vi "R1NH4SignalProcess.vi"(9 "error":errorcluster, 11 "LabVIEW Web Service":refnum<class "Web Service.lvclass">) -> (1 "error out":errorcluster)   [LabVIEW 2016]
uses:
  <vilib>/wsapi/Web Service.lvclass
  Controls/Tri State Control.ctl
  Controls/ISE_CF.ctl
panel:
  out "R1Na":T2 {"Steady State?" items=["False", "True", "NaN", ""]}
  out "Carousel Array":dbl[][](array[numeric])
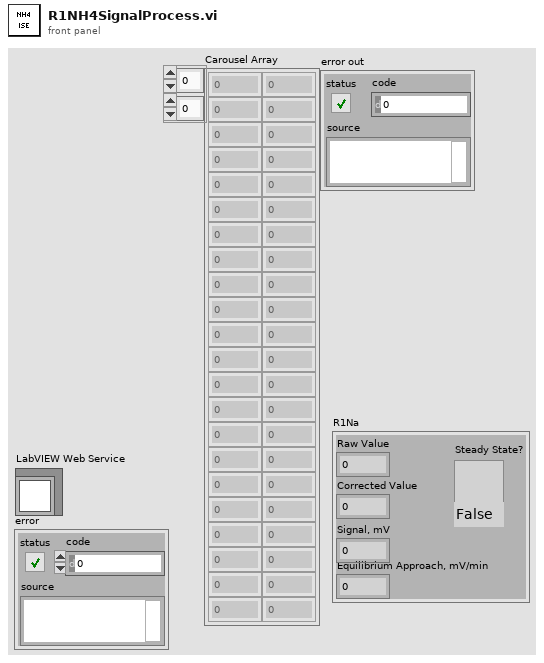
[diagram p1: front panel]
types:
  T1 = typedef "Tri State Control.ctl" = u16
  T2 = cluster{"Raw Value":dbl, "Corrected Value":dbl, "Signal, mV":dbl, "Equilibrium Approach, mV/min":dbl, "Steady State?":T1}
  T3 = typedef "ISE_CF.ctl" = cluster{"Correction Factor":dbl, "Ion":string, "Correct For Ion?":bool}
  T4 = cluster{"Equil Approach Set point, mV/min":dbl, "Equil Approach dt, s":dbl, "Interference Correction Factors":T3[], "Detect Equilibrium?":bool, "Probe Intercept":dbl, "Probe Slope":dbl, "Baseline":dbl, "Detection Limit, M":dbl}
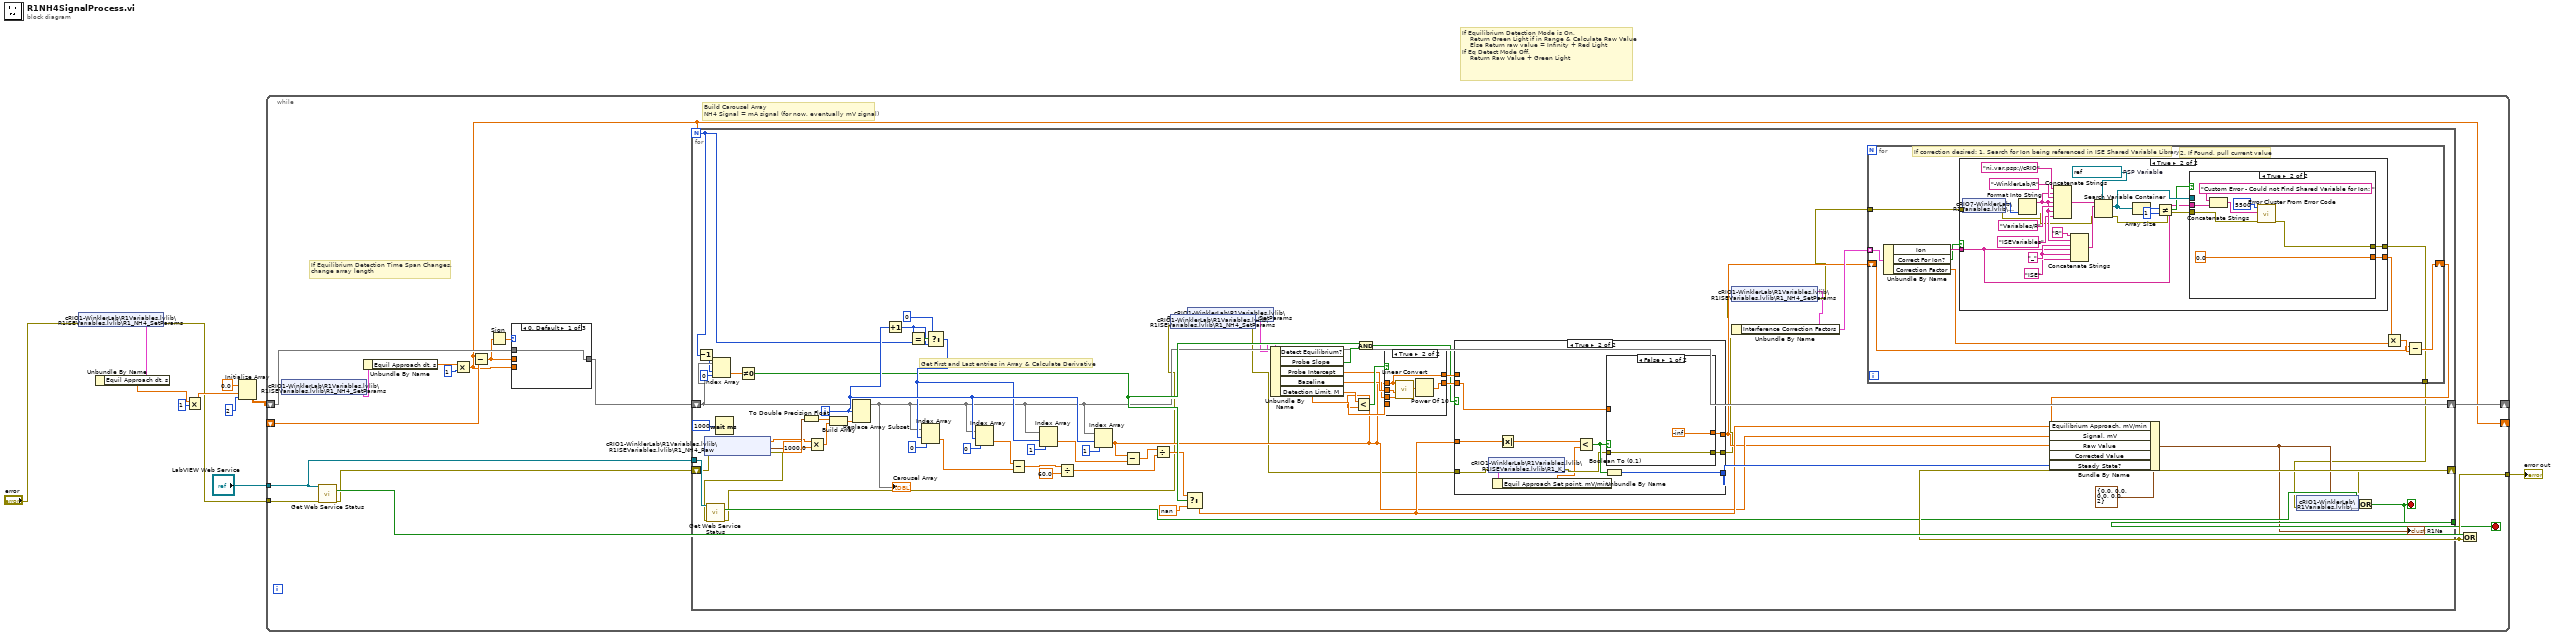
[diagram p0: block diagram]
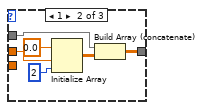
[diagram p2: hidden frame]
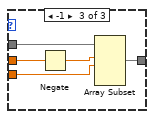
[diagram p3: hidden frame]
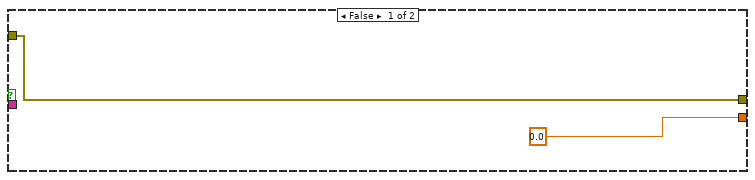
[diagram p4: hidden frame]
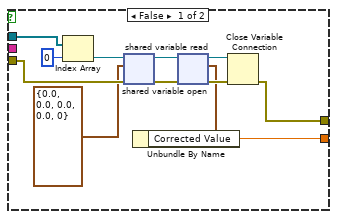
[diagram p5: hidden frame]
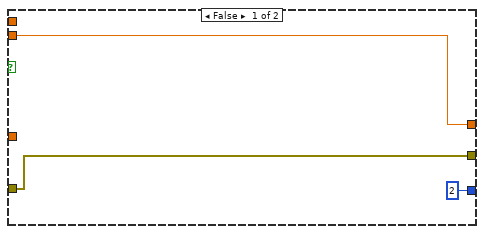
[diagram p7: hidden frame]
diagram:
  # "If Equilibrium Detection Mode is On, \n    Return Green Light if in Range & Calculate Raw Value\n    Else Return raw value = Infinity + Red Light\nIf Eq Detect Mode Off,\n    Return Raw Value + Green Light"
  n1 = shared-variable "cRIO1-WinklerLab\\R1Variables.lvlib\\R1ISEVariables.lvlib\\R1_NH4_SetParams"(error in="error") -> (w5:T4, error out=w1:errorcluster)
  n2 = Unbundle By Name(w5) -> ("Equil Approach dt, s"=w4:dbl)
  n3 = Multiply(x=w4, y=1) -> (x*y=w3:dbl)
  n4 = Initialize Array(0.0 ("element"), w3, 2 ("dimension size")) -> (w7:dbl[][])
  n5 = while {
    tunnel: "LabVIEW Web Service" -> [w27]
    tunnel: w1 -> [w18]
    shift-right: [w21] -> _
    shift-left: w7 -> [w24]
    shift-right: [w12] -> _
    shift-left: _ -> [w20]
    tunnel: [w17] -> w6
    stop <- w16 stop-if-true
    # "Build Carousel Array\nNH4 Signal = mA signal (for now, eventually mV signal)"
    # "If Equilibrium Detection Time Span Changes, \nchange array length"
    n6 = shared-variable "cRIO1-WinklerLab\\R1Variables.lvlib\\R1ISEVariables.lvlib\\R1_NH4_SetParams"() -> (w13:T4)  [unwired: 1 in, 1 out]
    n7 = call <vilib>:"Get Web Service Status.vi"("LabVIEW Web Service"=w27, "error in (no error)"=w18) -> ("service stopping?"=w19:bool, "error out"=w15:errorcluster)  [unwired: 11 in, 1 out]
    n8 = Unbundle By Name(w13) -> ("Equil Approach dt, s"=w14:dbl)
    n9 = Multiply(x=w14, y=1) -> (x*y=w12:dbl)
    n10 = Subtract(x=w12, y=w20) -> (x-y=w23:dbl)
    n11 = Sign(1:w23) -> (0:w25:dbl)
    n12 = case shown="0, Default" w25 {
      tunnel: w24 -> [w28 w32 w35]
      tunnel: w23 -> [_ w29 w37]
      tunnel: [w28 w30 w39] -> w22
      tunnel: w12 -> [_ _ w38]
      frame 0, Default {
      }
      frame 1 {
        n13 = Initialize Array(0.0 ("element"), w29, 2 ("dimension size")) -> (w31:dbl[][])
        n14 = Build Array (concatenate)(w32, w31) -> (w30:dbl[][])
      }
      frame -1 {
        n15 = Negate(x=w37) -> (-x=w36:dbl)
        n16 = Array Subset(array=w35, index (row)=w36, length (row)=w38) -> (w39:dbl[][])  [unwired: 2 in]
      }
    }
    n17 = for {
      N: w12 -> [w79]
      tunnel: w27 -> [w101]
      shift-right: [w74] -> w21
      shift-left: w22 -> [w85]
      shift-right: [w51] -> w17
      shift-left: w15 -> [w67]
      tunnel: [w66] -> w16
      i -> [w90]
      stop <- w66 stop-if-true
      # "Get First and Last entries in Array & Calculate Derivative"
      n18 = Decrement(x=w79) -> (x-1=w80:i32)
      n19 = shared-variable "cRIO1-WinklerLab\\R1Variables.lvlib\\R1ISEVariables.lvlib\\R1_NH4_Raw"(error in=w67) -> (w63:dbl, error out=w76:errorcluster, w77:timestamp)
      n20 = call <vilib>:"Get Web Service Status.vi"("LabVIEW Web Service"=w101, "error in (no error)"=w76) -> ("service stopping?"=w78:bool, "error out"=w43:errorcluster)  [unwired: 11 in, 1 out]
      n21 = Index Array(array=w85, index (row)=w80, index (col)=0 ("disabled index (col)")) -> (element=w83:dbl)
      n22 = Wait (ms)(milliseconds to wait=u32 1000) -> ()  [unwired: 1 out]
      n23 = Not Equal To 0?(x=w83) -> (x != 0?=w82:bool)
      n24 = To Double Precision Float(number=w77) -> (double precision float=w100:dbl)
      n25 = Multiply(x=w63, y=1000.0) -> (x*y=w62:dbl)
      n26 = Build Array(w100, w62) -> (w99:dbl[])
      n27 = Replace Array Subset(array=w85, new element=w99, index (row)=w90) -> (w74:dbl[][])  [unwired: 1 in]
      "Carousel Array" <- w74
      n28 = Increment(x=w90) -> (x+1=w60:i32)
      n29 = Equal?(x=w60, y=w79) -> (x = y?=w87:bool)
      n30 = Select(t=0, s=w87, f=w60) -> (s? t:f=w86:i32)
      n31 = Index Array(array=w74, index (row)=w86, index (col)=0 ("disabled index (col)")) -> (element=w92:dbl)
      n32 = Index Array(array=w74, index (row)=w90, index (col)=0 ("disabled index (col)")) -> (element=w88:dbl)
      n33 = Subtract(x=w88, y=w92) -> (x-y=w57:dbl)
      n34 = Index Array(array=w74, index (row)=w86, index (col)=1 ("disabled index (col)")) -> (element=w91:dbl)
      n35 = Divide(x=w57, y=60.0) -> (x/y=w56:dbl)
      n36 = Index Array(array=w74, index (row)=w90, index (col)=1 ("disabled index (col)")) -> (element=w52:dbl)
      n37 = Subtract(x=w52, y=w91) -> (x-y=w97:dbl)
      n38 = Divide(x=w97, y=w56) -> (x/y=w73:dbl)
      n39 = shared-variable "cRIO1-WinklerLab\\R1Variables.lvlib\\R1ISEVariables.lvlib\\R1_NH4_SetParams"(error in=w43) -> (w45:T4, error out=w44:errorcluster)
      n40 = Select(t=w73, s=w82, f=nan) -> (s? t:f=w54:dbl)
      n41 = shared-variable "cRIO1-WinklerLab\\R1Variables.lvlib\\R1ISEVariables.lvlib\\R1_NH4_SetParams"() -> ()  [unwired: 1 in, 2 out]
      n42 = Unbundle By Name(w45) -> ("Detect Equilibrium?"=w75:bool, "Probe Slope"=w71:dbl, "Probe Intercept"=w53:dbl, "Baseline"=w61:dbl, "Detection Limit, M"=w65:dbl)
      n43 = Less?(x=w61, y=w52) -> (x < y?=w72:bool)
      n44 = And(x=w82, y=w75) -> (x .and. y?=w68:bool)
      n45 = case shown="True" w72 {
        tunnel: w71 -> [_ w161]
        tunnel: w53 -> [_ w160]
        tunnel: w52 -> [w156 w159]
        tunnel: [w155 w158] -> w70
        tunnel: [w156 w159] -> w69
        tunnel: w65 -> [w155 _]
        frame False {
        }
        frame True {
          n46 = call "Linear Convert.vi"("Intercept"=w160, "Slope"=w161, "Signal"=w159) -> ("Result"=w157:dbl)  [unwired: 8 in]
          n47 = Power Of 10(x=w157) -> (10^x=w158:dbl)
        }
      }
      n48 = case shown="True" w68 {
        tunnel: [w164 w175] -> w48
        tunnel: w54 -> [_ w174]
        tunnel: [i16 2 w172] -> w89
        tunnel: w44 -> [w163 w168]
        tunnel: [w163 w169] -> w42
        tunnel: w70 -> [w164 w170]
        tunnel: w69 -> [_ _]
        frame False {
        }
        frame True {
          n49 = shared-variable "cRIO1-WinklerLab\\R1Variables.lvlib\\R1ISEVariables.lvlib\\R1_K_SetParams"(error in=w168) -> (w165:T4, error out=w167:errorcluster)
          n50 = Unbundle By Name(w165) -> ("Equil Approach Set point, mV/min"=w166:dbl)
          n51 = Absolute Value(x=w174) -> (abs(x)=w171:dbl)
          n52 = Less?(x=w171, y=w166) -> (x < y?=w173:bool)
          n53 = Boolean To (0,1)(Boolean=w173) -> (0, 1=w172:i16)
          n54 = case shown="False" w173 {
            tunnel: [-inf w178] -> w175
            tunnel: w167 -> [w177 w179]
            tunnel: [w177 w179] -> w169
            tunnel: w170 -> [_ w178]
            frame False {
            }
            frame True {
            }
          }
        }
      }
      n55 = shared-variable "cRIO1-WinklerLab\\R1Variables.lvlib\\R1ISEVariables.lvlib\\R1_NH4_SetParams"(error in=w42) -> (w40:T4, error out=w41:errorcluster)
      n56 = Unbundle By Name(w40) -> ("Interference Correction Factors"=w49:T3[])
      n57 = for {
        tunnel: w49 -> [w111] mode=indexing
        tunnel: w41 -> [w110]
        shift-right: [w103] -> w47
        shift-left: w48 -> [w104]
        tunnel: [w102] -> w46
        # "2. If Found, pull current value"
        # "If correction desired: 1. Search for Ion being referenced in ISE Shared Variable Library"
        n58 = Unbundle By Name(w111) -> ("Ion"=w109:string, "Correct For Ion?"=w108:bool, "Correction Factor"=w106:dbl)
        n59 = case shown="True" w108 {
          tunnel: w110 -> [w113 w120]
          tunnel: w109 -> [_ w117]
          tunnel: [0.0 ("Corrected Value") w115] -> w107
          tunnel: [w113 w114] -> w102
          frame False {
          }
          frame True {
            w116 = refnum<k21> refnum  # PSP Variable
            w133 = "_" ("string")
            n60 = shared-variable "cRIO7-WinklerLab\\R1Variables.lvlib\\R1OtherConstants.lvlib\\R1No"(error in=w120) -> (w134:i16, error out=w119:errorcluster)
            n61 = Format Into String(w134) -> (resulting string=w128:string)  [unwired: 3 in, 1 out]
            n62 = Concatenate Strings("ni.var.psp://cRIO", w128, "-WinklerLab/R" ("string"), w128, "Variables/R" ("string"), w128, "ISEVariables" ("string")) -> (w126:string)
            n63 = Concatenate Strings("R" ("string"), w128, w133, w117, w133, "ISE" ("string")) -> (w125:string)
            n64 = Search Variable Container(7:w116, 8:w119, 10:w125, 11:w126) -> (0:w118:errorcluster, 2:w122:refnum<k21>[])  [unwired: 2 in, 1 out]
            n65 = Array Size(array=w122) -> (size(s)=w124:i32)
            n66 = Not Equal?(x=w124, y=1) -> (x != y?=w121:bool)
            n67 = case shown="True" w121 {
              tunnel: w122 -> [w147 _]
              tunnel: w118 -> [w144 w154]
              tunnel: w117 -> [_ w152]
              tunnel: [w138 w151] -> w114
              tunnel: [w136 0.0 ("Corrected Value")] -> w115
              frame False {
                n68 = Index Array(array=w147, index=0) -> (element=w145:refnum<k21>)
                n69 = shared-variable-open(w145, w144, T2 {"Raw Value"=0.0, "Corrected Value"=0.0, "Signal, mV"=0.0, "Equilibrium Approach, mV/min"=0.0, "Steady State?"=0} ("ISE")) -> (w142:refnum<k21>, w139:errorcluster)  [unwired: 1 in]
                n70 = shared-variable-read(w142, w139) -> (w140:refnum<k21>, w141:errorcluster, w137:T2)  [unwired: 1 out]
                n71 = Unbundle By Name(w137) -> ("Corrected Value"=w136:dbl)
                n72 = Close Variable Connection(8:w141, 11:w140) -> (0:w138:errorcluster)
              }
              frame True {
                n73 = Concatenate Strings("Custom Error - Could not Find Shared Variable for Ion: " ("string"), w152) -> (w150:string)
                n74 = call <vilib>:"Error Cluster From Error Code.vi"("error in (no error)"=w154, "error message (\"\")"=w150, "error code (0)"=5500) -> ("error out"=w151:errorcluster)  [unwired: 6 in]
              }
            }
          }
        }
        n75 = Multiply(x=w107, y=w106) -> (x*y=w105:dbl)
        n76 = Subtract(x=w104, y=w105) -> (x-y=w103:dbl)
      }
      n77 = Bundle By Name(cluster=T2 {"Raw Value"=0.0, "Corrected Value"=0.0, "Signal, mV"=0.0, "Equilibrium Approach, mV/min"=0.0, "Steady State?"=2} ("R1NH4"), "Equilibrium Approach, mV/min"=w54, "Signal, mV"=w52, "Raw Value"=w48, "Corrected Value"=w47, "Steady State?"=w89) -> (w50:T2)
      "R1Na" <- w50
      n78 = shared-variable "cRIO1-WinklerLab\\R1Variables.lvlib\\R1ISEVariables.lvlib\\R1_NH4_ISE"(w50, error in=w46) -> (error out=w51:errorcluster)
      n79 = Or(x=w78, y=w51) -> (x .or. y?=w66:bool)
    }
    n80 = Or(x=w19, y=w17) -> ()  [unwired: 1 out]
  }
  "error out" <- w6
